vi "Unit Test - copy but skip if exist.vi"() -> (3 "Array":T1(array[cluster])=[{"state"="Idle", "error out"={"status"=FALSE, "code"=0, "source"=""}, "Execution:State"=enum."Idle"}, {"state"="CSM Documentation", "error out"={"status"=FALSE, "code"=0, "source"=""}, "Execution:State"=enum."Idle"}, {"state"="VI Reference", "error out"={"status"=FALSE, "code"=0, "source"=""}, "Execution:State"=enum."Idle"}, {"state"="Error Handler", "error out"={"status"=FALSE, "code"=0, "source"=""}, "Execution:State"=enum."Bad"}, {"state"="Critical Error", "error out"={"status"=FALSE, "code"=0, "source"=""}, "Execution:State"=enum."Idle"}, {"state"="Target Timeout Error", "error out"={"status"=FALSE, "code"=0, "source"=""}, "Execution:State"=enum."Idle"}, {"state"="Target Error", "error out"={"status"=FALSE, "code"=0, "source"=""}, "Execution:State"=enum."Idle"}, {"state"="Async Response", "error out"={"status"=FALSE, "code"=0, "source"=""}, "Execution:State"=enum."Idle"}, {"state"="Response", "error out"={"status"=FALSE, "code"=0, "source"=""}, "Execution:State"=enum."Idle"}, {"state"="Async Message Posted", "error out"={"status"=FALSE, "code"=0, "source"=""}, "Execution:State"=enum."Idle"}, {"state"="Initialize Core Data", "error out"={"status"=FALSE, "code"=0, "source"=""}, "Execution:State"=enum."Idle"}, {"state"="Exit", "error out"={"status"=FALSE, "code"=0, "source"=""}, "Execution:State"=enum."Idle"}, {"state"="Data: Initialize", "error out"={"status"=FALSE, "code"=0, "source"=""}, "Execution:State"=enum."Idle"}, {"state"="Data: Update Indicators", "error out"={"status"=FALSE, "code"=0, "source"=""}, "Execution:State"=enum."Idle"}, {"state"="Data: Cleanup", "error out"={"status"=FALSE, "code"=0, "source"=""}, "Execution:State"=enum."Idle"}, {"state"="Macro: Initialize", "error out"={"status"=FALSE, "code"=0, "source"=""}, "Execution:State"=enum."Idle"}, {"state"="Macro: Exit", "error out"={"status"=FALSE, "code"=0, "source"=""}, "Execution:State"=enum."Idle"}, {"state"="API: API1", "error out"={"status"=FALSE, "code"=0, "source"=""}, "Execution:State"=enum."Idle"}, {"state"="API: API2", "error out"={"status"=FALSE, "code"=0, "source"=""}, "Execution:State"=enum."Idle"}, {"state"="Action: action1", "error out"={"status"=FALSE, "code"=0, "source"=""}, "Execution:State"=enum."Idle"}, {"state"="Action: action2", "error out"={"status"=FALSE, "code"=0, "source"=""}, "Execution:State"=enum."Idle"}])   [LabVIEW 2017, in "testcase-csmhelper.lvclass"]
uses:
  testcase-csmhelper.lvclass
  src/user.lib/_NEVSTOP/Communicable State Machine(CSM)/_csmHelper/CSM-Helper.lvclass/CSM-Helper.ctl
  src/user.lib/_NEVSTOP/Communicable State Machine(CSM)/_csmHelper/Properties/Read VI Ref.vi
  src/user.lib/_NEVSTOP/Communicable State Machine(CSM)/_csmHelper/API/Create From VI Reference.vi
  src/user.lib/_NEVSTOP/Communicable State Machine(CSM)/_csmHelper/Properties/Read States.vi
  src/user.lib/_NEVSTOP/Communicable State Machine(CSM)/_csmHelper/API/Start Undo.vi
  src/user.lib/_NEVSTOP/Communicable State Machine(CSM)/_csmHelper/API/Copy State.vi
  src/user.lib/_NEVSTOP/Communicable State Machine(CSM)/_csmHelper/API/Stop Undo.vi
  src/user.lib/_NEVSTOP/Communicable State Machine(CSM)/_csmHelper/API/Undo.vi
  src/user.lib/_NEVSTOP/Communicable State Machine(CSM)/_csmHelper/API/Destroy.vi
  src/user.lib/_NEVSTOP/Communicable State Machine(CSM)/_csmHelper/CSM-Helper.lvclass
  src/user.lib/_NEVSTOP/Communicable State Machine(CSM)/_csmHelper/API/Open Block Diagram.vi
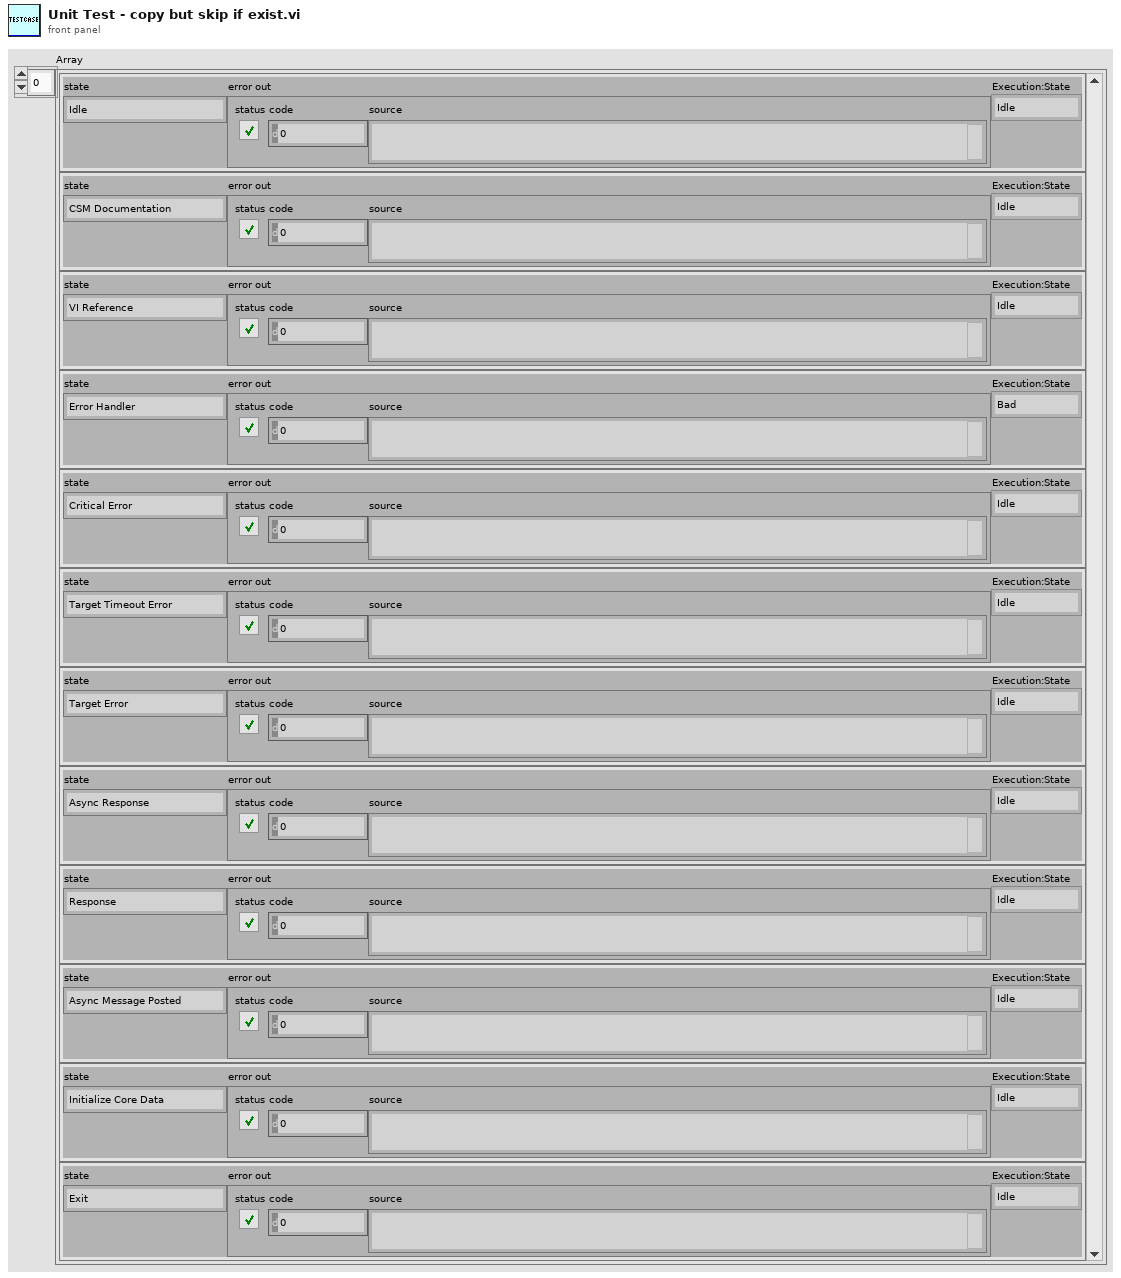
[diagram p1: front panel]
types:
  T1 = cluster{"state":string, "error out":errorcluster, "Execution:State":enum32{"Bad", "Idle", "Run top level", "Running"}}[]
  T2 = enum32{"Bad", "Idle", "Run top level", "Running"}
  T3 = cluster{string, "error out":errorcluster, "Exec.State":enum32{"Bad", "Idle", "Run top level", "Running"}}
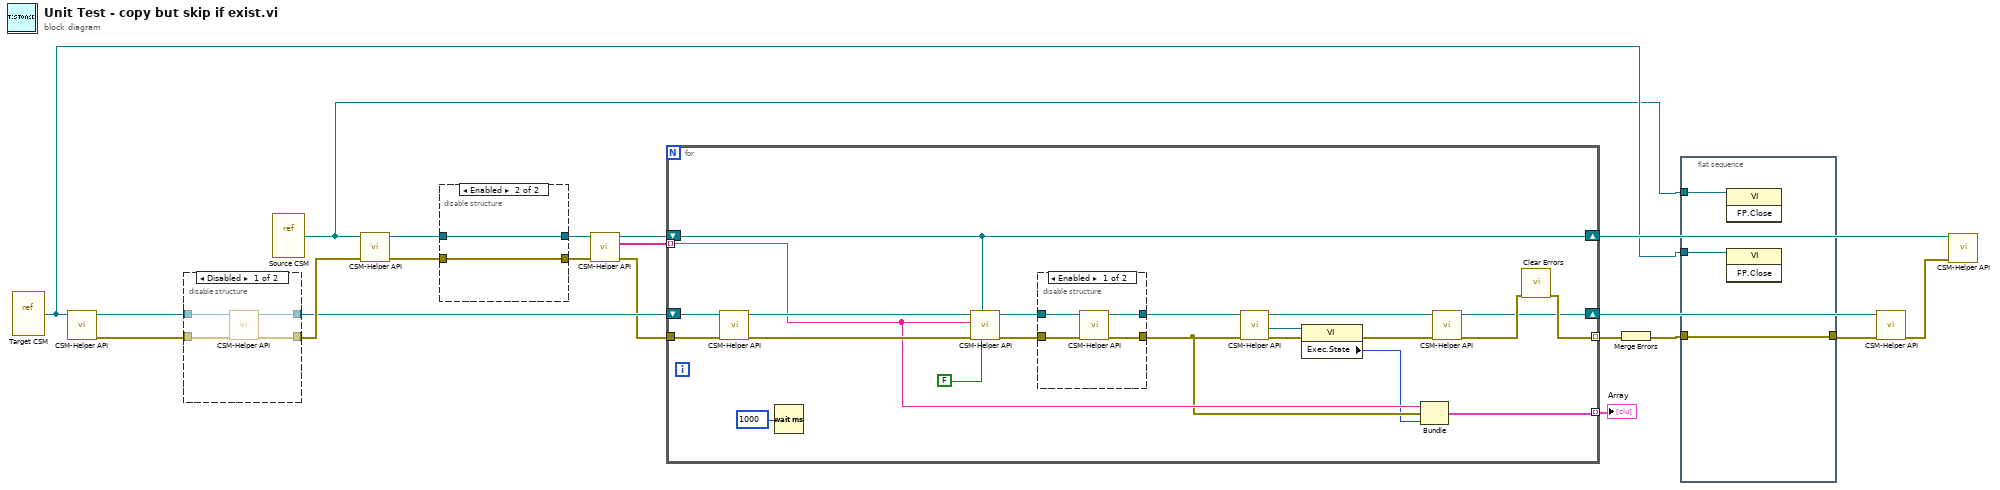
[diagram p0: block diagram]
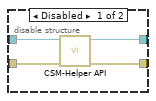
[diagram p3: hidden frame]
diagram:
  n1 = vi-ref "Target CSM.vi"() -> (w2:refnum<vi>)
  n2 = call-poly "CSM-Helper API.vi"("VI"=w2) -> ("error out"=w18:errorcluster, "CSM-Helper.lvclass"=w17:refnum<class "CSM-Helper.lvclass">)  [unwired: 9 in]
  n3 = disable-structure shown="Disabled" {
    disable-tunnel: w18 -> [w24 w25]
    disable-tunnel: w17 -> [w23 w26]
    disable-tunnel: [w22 w25] -> w12
    disable-tunnel: [w21 w26] -> w11
    frame Disabled {
      n4 = call-poly "CSM-Helper API.vi"("error in (no error)"=w24, "CSM-Helper in"=w23) -> ("error out"=w22:errorcluster, "CSM-Helper out"=w21:refnum<class "CSM-Helper.lvclass">)  [unwired: 8 in]
    }
    frame Enabled {
    }
  }
  n5 = vi-ref "Source CSM.vi"() -> (w1:refnum<vi>)
  n6 = call-poly "CSM-Helper API.vi"("error in (no error)"=w12, "VI"=w1) -> ("error out"=w15:errorcluster, "CSM-Helper.lvclass"=w16:refnum<class "CSM-Helper.lvclass">)  [unwired: 8 in]
  n7 = disable-structure shown="Enabled" {
    disable-tunnel: w16 -> [w30 w31]
    disable-tunnel: w15 -> [w29 w32]
    disable-tunnel: [w28 w32] -> w14
    disable-tunnel: [w27 w31] -> w13
    frame Disabled {
      n8 = call-poly "CSM-Helper API.vi"("error in (no error)"=w29, "CSM-Helper in"=w30) -> ("error out"=w28:errorcluster, "CSM-Helper out"=w27:refnum<class "CSM-Helper.lvclass">)  [unwired: 8 in]
    }
    frame Enabled {
    }
  }
  n9 = call-poly "CSM-Helper API.vi"("error in (no error)"=w14, "CSM-Helper in"=w13) -> ("error out"=w10:errorcluster, "Value"=w6:string[], "CSM-Helper out"=w9:refnum<class "CSM-Helper.lvclass">)  [unwired: 7 in]
  n10 = for {
    shift-right: [w41] -> w20
    shift-left: w11 -> [w52]
    shift-right: [w47] -> w7
    shift-left: w9 -> [w47]
    tunnel: w6 -> [w45] mode=indexing
    tunnel: w10 -> [w51]
    tunnel: [w46] -> w19 mode=indexing
    tunnel: [w44] -> w5 mode=indexing
    n11 = call-poly "CSM-Helper API.vi"("error in (no error)"=w51, "CSM-Helper in"=w52) -> ("error out"=w50:errorcluster, "CSM-Helper out"=w49:refnum<class "CSM-Helper.lvclass">)  [unwired: 8 in]
    n12 = Wait (ms)(milliseconds to wait=u32 1000) -> ()  [unwired: 1 out]
    n13 = call-poly "CSM-Helper API.vi"("Already Exist Action:\nReplace(T) / Skip(F)"=FALSE ("Already Exist Action:\nReplace(T) / Skip(F)"), "SourceCSM"=w47, "error in (no error)"=w50, "Case"=w45, "CSM-Helper.lvclass"=w49) -> ("error out"=w48:errorcluster, "CSM-Helper out 2"=w53:refnum<class "CSM-Helper.lvclass">)  [unwired: 5 in]
    n14 = disable-structure shown="Enabled" {
      disable-tunnel: [w57 w59] -> w39
      disable-tunnel: w48 -> [w56 w58]
      disable-tunnel: [w55 w58] -> w40
      disable-tunnel: w53 -> [w54 w59]
      frame Enabled {
        n15 = call-poly "CSM-Helper API.vi"("error in (no error)"=w56, "CSM-Helper in"=w54) -> ("error out"=w55:errorcluster, "CSM-Helper out"=w57:refnum<class "CSM-Helper.lvclass">)  [unwired: 8 in]
      }
      frame Disabled {
      }
    }
    n16 = call-poly "CSM-Helper API.vi"("error in (no error)"=w40, "CSM-Helper in"=w39) -> ("error out"=w37:errorcluster, "VI"=w35:refnum<vi>, "CSM-Helper out"=w38:refnum<class "CSM-Helper.lvclass">)  [unwired: 7 in]
    n17 = property class="VI"(reference=w35, error in=w37) -> (error out=w36:errorcluster, "Exec.State"=w34:T2)  [unwired: 1 out]
    n18 = Bundle(w45, "error out"=w40, "Exec.State"=w34) -> (w44:T3)  [unwired: 1 in]
    n19 = call-poly "CSM-Helper API.vi"("error in (no error)"=w36, "CSM-Helper in"=w38) -> ("error out"=w42:errorcluster, "CSM-Helper out"=w41:refnum<class "CSM-Helper.lvclass">)  [unwired: 8 in]
    n20 = call <vilib>:"Clear Errors.vi"("error in (no error)"=w42) -> ("error out"=w46:errorcluster)  [unwired: 5 in, 1 out]
  }
  "Array" <- w5
  n21 = Merge Errors(w19) -> (w4:errorcluster)
  n22 = flat-sequence {
    tunnel: [w62] -> w3
    tunnel: w4 -> [w62]
    tunnel: w2 -> [w61]
    tunnel: w1 -> [w60]
    frame #0 {
      n23 = invoke class="VI" method="FP.Close"(reference=w60) -> ()  [unwired: 2 in, 3 out]
      n24 = invoke class="VI" method="FP.Close"(reference=w61) -> ()  [unwired: 2 in, 3 out]
    }
  }
  n25 = call-poly "CSM-Helper API.vi"("error in (no error)"=w3, "CSM-Helper in"=w20) -> ("error out"=w8:errorcluster)  [unwired: 8 in, 1 out]
  n26 = call-poly "CSM-Helper API.vi"("error in (no error)"=w8, "CSM-Helper in"=w7) -> ()  [unwired: 8 in, 2 out]
